vi "Pointer.Duration.vi"() -> ()   [LabVIEW 2016]
uses:
  <vilib>/Platform/TimedLoop/XDataNode/timing_clust.ctl
  <vilib>/Platform/TimedLoop/XDataNode/nitl_modes.ctl
  <vilib>/Platform/TimedLoop/XDataNode/wakeup.ctl
  Source/Classes/Pointer/Memory.Pointer.lvclass/Memory.Pointer.ctl
  Source/Classes/Pointer/Memory.Pointer.Read.Safe.1D.U8.vi
  Source/Classes/Pointer/Memory.Pointer.Read.Unsafe.1D.U8.vi
  Source/Classes/Pointer/Memory.Pointer.Parameter Check.Null Pointer.vi
  Source/Classes/Pointer/Memory.Pointer.Parameter Check.Subset.Power of 2.vi
  Source/Classes/Pointer/Memory.Pointer.Get Address.vi
  Source/Classes/Pointer/Memory.Pointer.Errors.vi
  Source/Classes/Pointer/Memory.Pointer.Errors.Null Pointer.vi
  Source/Classes/Pointer/Memory.Pointer.Errors.Out of Bounds.vi
  Source/Classes/Pointer/Memory.Pointer.Get Size.vi
  Source/VIs/Memory.Count to Size.Power of 2.vi
  Source/Classes/Pointer/Memory.Pointer.Errors.Create Error.vi
  Source/Submodules/SEH/Source/VIs/Static Error Handling.Source Buffer.Write.String.vi
  Source/Classes/Pointer/Memory.Pointer.Errors.Write Pointer Size.vi
  Source/Submodules/SEH/Source/VIs/Static Error Handling.Source Buffer.Write.Numeric.Scalar.Base10.vi
  Source/Submodules/SEH/Source/VIs/Static Error Handling.Source Buffer.Write.Numeric.Scalar.Base10 (U64).vi
  Source/Submodules/SEH/Source/VIs/Static Error Handling.Error Cluster Constant.vi
  Source/Submodules/SEH/Source/VIs/Static Error Handling.Error Cluster Constant (256B).vi
  Source/Submodules/SEH/Source/VIs/Static Error Handling.Parameters.Status.Set.vi
  Source/Submodules/SEH/Source/VIs/Static Error Handling.Parameters.Code.Set.vi
  Source/Submodules/SEH/Source/VIs/Static Error Handling.Parameters.VI Source.Set.vi
  Source/Constants/Memory.Constants.vi
  Source/Constants/Memory.Constants.Library Name.vi
  Source/Classes/Pointer/Memory.Pointer.Errors.Get Info.vi
  Source/Classes/Internal/Memory.Pointer.Internal.lvclass
  C:/Git/Sourcetree/DSF/Source/Submodules/Memory/Source/Classes/Pointer/Memory.Pointer.lvclass
  Source/Classes/Internal/Memory.Pointer.Internal.Allocate.vi
  <vilib>/platform/TimedLoop/XDataNode/XDataNode.xnode
  <vilib>/Platform/TimedLoop/XDataNode/XDNodeRunTimeDep.lvlib
  Source/Classes/Pointer/Memory.Pointer.lvclass
panel:
  out "error out":errorcluster
  out "size":i32
  out "dvr duration":dbl format="%.3ps"
  out "pointer duration":dbl format="%.3ps"
  in  "iterations":i32=10000000 format="%.0p"
  in  "processor":i32=-2
  in  "size":u64=1024 format="%d bytes"
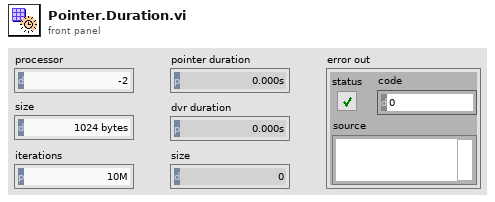
[diagram p1: front panel]
types:
  T1 = typedef "XDNodeRunTimeDep.lvlib/timing_clust.ctl" = cluster{"Expected End [f-1]":u64, "Actual End [f-1]":u64, "Finished Late? [f-1]":bool, "Expected End [i-1]":u64, "Actual End [i-1]":u64, "Finished Late? [i-1]":bool, "Expected Start [i]":u64, "Actual Start [i]":u64, "Expected Start [f]":u64, "Actual Start [f]":u64, "Source Name":string, "Structure Name":string, "Period":i64, "Deadline":i64, "Offset":i64, "Start":i64, "Priority":i32, "Timeout":i32, "Mode":T2, "Wakeup Reason":T3, "Error":errorcluster, "Source Type":string, "Secondary Source Type":string, "Global End Time":u64, "Global Start Time":u64, "Frame Duration":u64, "Iteration Duration":u64, "Assigned CPU":i32, "I/O Scan Engine Mode":u32}
  T2 = typedef "XDNodeRunTimeDep.lvlib/nitl_modes.ctl" = enum32{"No Change", "Process missed periods, maintain original phase", "Discard missed periods, maintain original phase", "Process missed periods, ignore original phase", "Discard missed periods, ignore original phase"}
  T3 = typedef "XDNodeRunTimeDep.lvlib/wakeup.ctl" = enum32{"Normal", "Aborted", "Asynchronous wakeup", "Timing source error", "Timed loop error", "Timeout"}
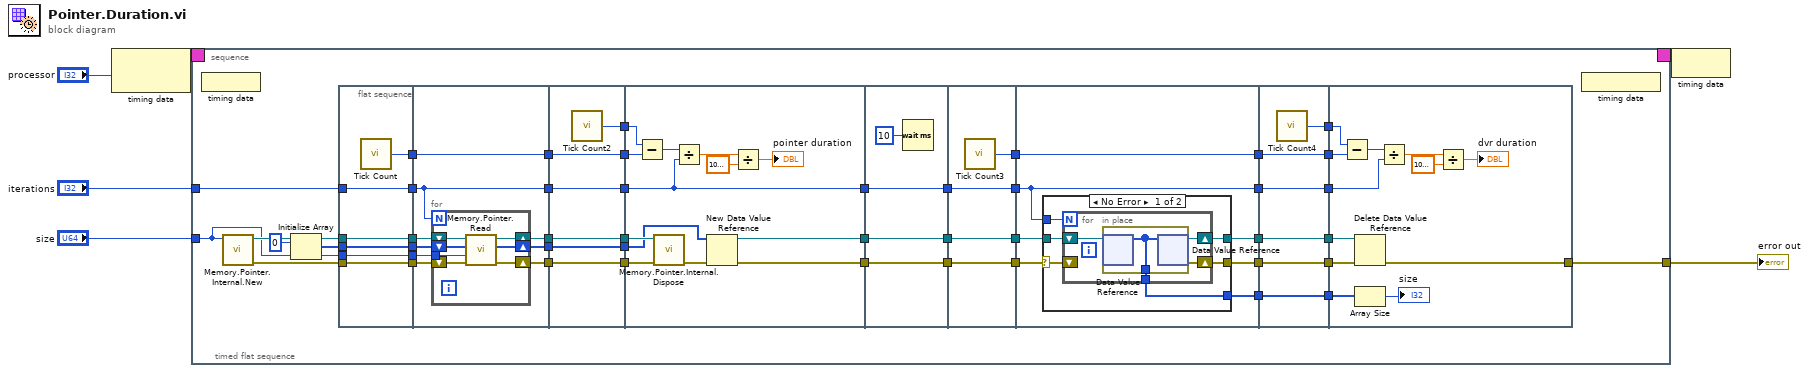
[diagram p0: block diagram]
diagram:
  n1 = node-c288("processor") -> (w6:T1)
  n2 = timed-sequence {
    timing: w6 -> [_]
    timing-out: [_] -> w5
    tunnel: "iterations" -> [w9]
    tunnel: "size" -> [w8]
    tunnel: [w7] -> w1
    n3 = timed-flat-sequence {
      tunnel: w9 -> [w12]
      tunnel: w8 -> [w10]
      tunnel: [w16] -> w7
      n4 = node-c288() -> ()  [unwired: 1 in]
      n5 = call "Memory.Pointer.Internal.New.vi"("size"=w10) -> ("error out"=w47:errorcluster, "pointer"=w48:refnum<class "Memory.Pointer.Internal.lvclass">)  [unwired: 9 in]
      n6 = Initialize Array(u8 0 ("element"), w10) -> (w42:u8[])
      n7 = flat-sequence {
        tunnel: [w60] -> w54
        tunnel: [w56] -> w53
        tunnel: [w59] -> w49
        tunnel: [w58] -> w46
        tunnel: [w57] -> w43
        tunnel: w12 -> [w60]
        tunnel: w48 -> [w59]
        tunnel: w47 -> [w58]
        tunnel: w42 -> [w57]
        tunnel: w10 -> [w55]
        tunnel: [w55] -> w11
        tunnel: w54 -> [w68]
        tunnel: w53 -> [w69]
        tunnel: [w69] -> w52
        tunnel: [w68] -> w51
        tunnel: w49 -> [w67]
        tunnel: w46 -> [w66]
        tunnel: [w65] -> w45
        tunnel: [w64] -> w44
        tunnel: w43 -> [w63]
        tunnel: [w62] -> w41
        tunnel: w11 -> [w61]
        tunnel: w52 -> [w78]
        tunnel: w51 -> [w82]
        tunnel: w45 -> [w81]
        tunnel: w44 -> [w80]
        tunnel: w41 -> [w79]
        tunnel: [w82] -> w40
        tunnel: [w81] -> w39
        tunnel: [w80] -> w38
        tunnel: [w79] -> w37
        tunnel: [w78] -> w36
        tunnel: [w77] -> w35
        tunnel: w40 -> [w83]
        tunnel: w39 -> [w92]
        tunnel: w38 -> [w93]
        tunnel: w37 -> [w86]
        tunnel: w36 -> [w91]
        tunnel: w35 -> [w90]
        tunnel: [w85] -> w34
        tunnel: [w84] -> w33
        tunnel: [w83] -> w25
        tunnel: w34 -> [w99]
        tunnel: w33 -> [w98]
        tunnel: [w99] -> w32
        tunnel: [w98] -> w31
        tunnel: [w96] -> w26
        tunnel: w25 -> [w96]
        tunnel: w32 -> [w103]
        tunnel: w31 -> [w102]
        tunnel: [w103] -> w30
        tunnel: [w102] -> w29
        tunnel: [w101] -> w28
        tunnel: [w100] -> w27
        tunnel: w26 -> [w100]
        tunnel: w30 -> [w108]
        tunnel: w29 -> [w109]
        tunnel: w28 -> [w110]
        tunnel: w27 -> [w105]
        tunnel: [w110] -> w24
        tunnel: [w107] -> w23
        tunnel: [w106] -> w19
        tunnel: [w105] -> w18
        tunnel: [w104] -> w14
        tunnel: w24 -> [w129]
        tunnel: w23 -> [w128]
        tunnel: [w129] -> w22
        tunnel: [w128] -> w21
        tunnel: [w127] -> w20
        tunnel: w19 -> [w126]
        tunnel: w18 -> [w125]
        tunnel: [w126] -> w17
        tunnel: [w125] -> w15
        tunnel: w14 -> [w124]
        tunnel: [w124] -> w13
        tunnel: w22 -> [w134]
        tunnel: w21 -> [w141]
        tunnel: w20 -> [w135]
        tunnel: w17 -> [w140]
        tunnel: [w133] -> w16
        tunnel: w15 -> [w132]
        tunnel: w13 -> [w131]
        frame #0 {
          n8 = call "Tick Count"() -> ("Tick Count(uSec)"=w56:u32)
        }
        frame #1 {
          n9 = for {
            N: w68 -> [_]
            shift-right: [w75] -> w64
            shift-left: w67 -> [w76]
            shift-right: [w71] -> w62
            shift-left: w63 -> [w72]
            shift-right: [w74] -> w65
            shift-left: w66 -> [w73]
            tunnel: w61 -> [w70]
            n10 = call-poly "Memory.Pointer.Read.vi"("error in (no error)"=w73, "offset (0)"=w70, "buffer in"=w72, "pointer in"=w76) -> ("error out"=w74:errorcluster, "buffer out"=w71:u8[], "pointer out"=w75:refnum<class "Memory.Pointer.Internal.lvclass">)  [unwired: 4 in, 1 out]
          }
        }
        frame #2 {
          n11 = call "Tick Count2"() -> ("Tick Count(uSec)"=w77:u32)
        }
        frame #3 {
          n12 = Subtract(x=w90, y=w91) -> (x-y=w89:u32)
          n13 = call "Memory.Pointer.Internal.Dispose.vi"("error in (no error)"=w92, "pointer"=w93) -> ("error out"=w87:errorcluster)  [unwired: 9 in]
          n14 = Divide(x=w89, y=w83) -> (x/y=w95:dbl)
          n15 = New Data Value Reference(data value=w86, error in=w87) -> (data value reference=w84:refnum<data-value>, error out=w85:errorcluster)
          n16 = Divide(x=w95, y=1000000.0) -> (x/y=→"pointer duration":dbl)
        }
        frame #4 {
          n17 = Wait (ms)(milliseconds to wait=u32 10) -> ()  [unwired: 1 out]
        }
        frame #5 {
          n18 = call "Tick Count3"() -> ("Tick Count(uSec)"=w101:u32)
        }
        frame #6 {
          n19 = case shown="No Error" w108 {
            selector: w108 -> [w114 w123]
            tunnel: w105 -> [w116 _]
            tunnel: w109 -> [w115 w122]
            tunnel: [w113 w123] -> w107
            tunnel: [w112 w122] -> w106
            tunnel: [w111 _] -> w104
            frame No Error {
              n20 = for {
                N: w116 -> [_]
                shift-right: [w119] -> w113
                shift-left: w114 -> [_]
                tunnel: [w117] -> w111
                shift-right: [w118] -> w112
                shift-left: w115 -> [w120]
                n21 = in-place {
                  in-place-border: [w121] -> w117
                  n22 = in-place-dvr #1(w120) -> (w121:u8[])  [unwired: 1 out]
                  n23 = in-place-dvr #1(w121) -> (w118:refnum<data-value>, w119:errorcluster)
                }
              }
            }
            frame Error {
            }
          }
        }
        frame #7 {
          n24 = call "Tick Count4"() -> ("Tick Count(uSec)"=w127:u32)
        }
        frame #8 {
          n25 = Subtract(x=w135, y=w134) -> (x-y=w137:u32)
          n26 = Delete Data Value Reference(data value reference=w140, error in=w141) -> (error out=w133:errorcluster)  [unwired: 1 out]
          n27 = Array Size(array=w131) -> (size(s)=→"size":i32)
          n28 = Divide(x=w137, y=w132) -> (x/y=w139:dbl)
          n29 = Divide(x=w139, y=1000000.0) -> (x/y=→"dvr duration":dbl)
        }
      }
      n30 = node-c288() -> ()  [unwired: 1 out]
    }
  }
  "error out" <- w1
  n31 = node-c288(w5) -> ()
